vi "setSweepTable.vi"(8 "error in (no error)":errorcluster, 9 "Table(s)":variant, 10 "Channel(s)":variant, 11 "Instrument.LockinAPI in":refnum<class "Instrument.LockinAPI.lvclass">) -> (0 "error out":errorcluster, 3 "Instrument.LockinAPI out":refnum<class "Instrument.LockinAPI.lvclass">)   [LabVIEW 2019, in "Instrument.LockinAPI.lvclass"]
doc: "API to set Sweep Waveform"
uses:
  Instrument.LockinAPI.lvclass
  C:/Users/patrick/Documents/GitHub/Instrument-Framework/lvsrc/Framework/Instrument/Instrument.lvclass
  Typedefs/LockinAPI.Commands--Enum.ctl
  <vilib>/Utility/Data Type/NI_Data Type.lvlib
  Instrument/Instrument.lvclass
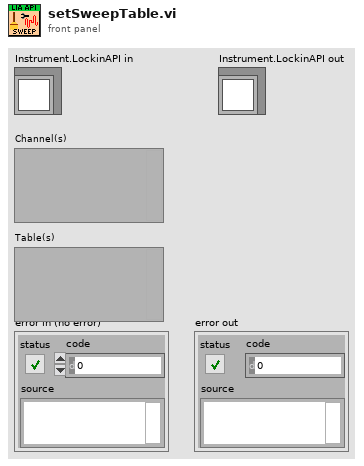
[diagram p1: front panel]
types:
  T1 = cluster{"Sweep Time (s)":dbl, "Initial Wait (s)":dbl, "Return to Start":bool, "Channels":cluster{"Enable?":bool, "Channel":u16, "Start":dbl, "End":dbl, "Pattern":enum16{"Ramp /", "Ramp /\\", "Smooth Ramp _/", "Smooth Ramp _/\\_", "Table"}, "Table":dbl[]}[]}
  T2 = typedef "Instrument.LockinAPI.lvclass/LockinAPI.Commands--Enum.ctl" = enum16{"setAI", "setAO", "setAO_Amplitude", "setAO_DC", "setAO_Frequency", "setAO_Phase", "setAO_Function", "setAO_I+", "setREF", "setREF_Frequency", "setREF_Phase", "setREF_TC", "setREF_Roll-Off", "setDAQ", "setSampling", "setOffset", "setState", "getState", "getAO", "getAI", "getResults", "getSampling", "getAOconfig", "getREFconfig", "setInputGain", "setOutputGain", "getInputGain", "getOutputGain", "setSamplingMode", "getSamplingMode", "setSweep", "setSweepTime", "setSweepTable", "getStatus", "getSweepResults", "getSweepWaveforms", "startSweep", "stopSweep", "setAUX", "getAUX"}
  T3 = cluster{"Enable?":bool, "Channel":u16, "Start":dbl, "End":dbl, "Pattern":enum16{"Ramp /", "Ramp /\\", "Smooth Ramp _/", "Smooth Ramp _/\\_", "Table"}, "Table":dbl[]}[]
  T4 = typedef "NI_Data Type.lvlib/Data Type.ctl" = enum8{"Invalid Type", "Void", "I8", "I16", "I32", "I64", "U8", "U16", "U32", "U64", "Single Float", "Double Float", "Extended Float", "Single Complex", "Double Complex", "Extended Complex", "Enum U8", "Enum U16", "Enum U32", "Enum U64", "Single Float With Unit", "Double Float With Unit", "Extended Float With Unit", "Single Complex with Unit", "Double Complex with Unit", "Extended Complex with Unit", "Boolean", "String", "Path", "Picture", "Tag", "Array", "Cluster", "Variant", "LV Variant", "Waveform", "Timestamp", "Digital Waveform", "Digital Data", "ExpressData", "Refnum", "External Data", "VI", "Poly VI", "LabVIEW Class Instance", "Fixed Point", "Set Collection", "Map Collection"}
  T5 = cluster{"Enable?":bool, "Channel":u16, "Start":dbl, "End":dbl, "Pattern":enum16{"Ramp /", "Ramp /\\", "Smooth Ramp _/", "Smooth Ramp _/\\_", "Table"}, "Table":dbl[]}
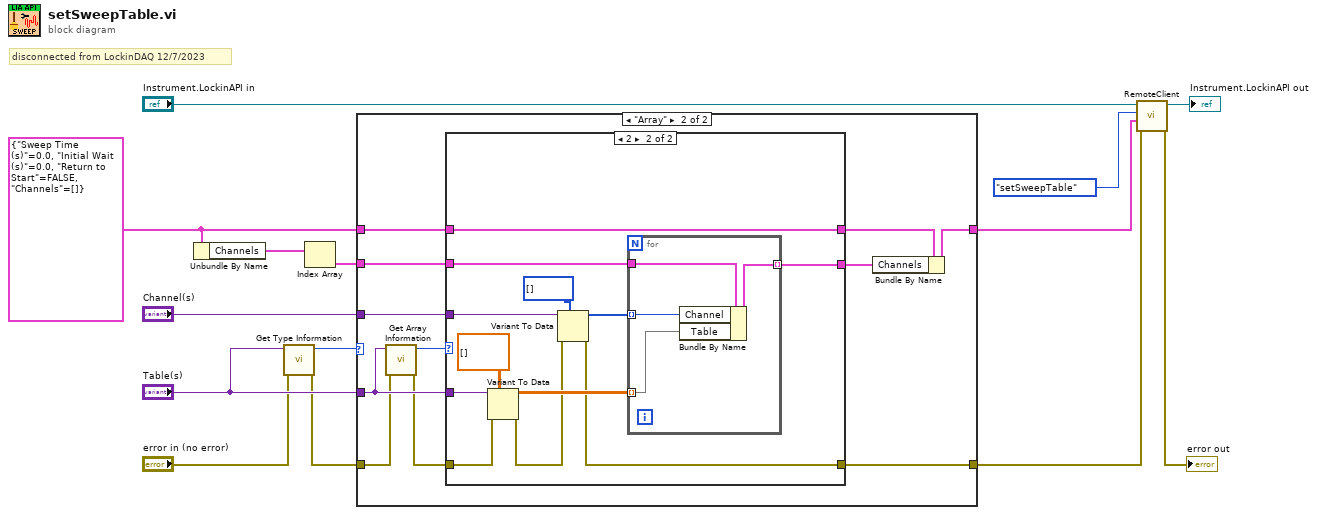
[diagram p0: block diagram]
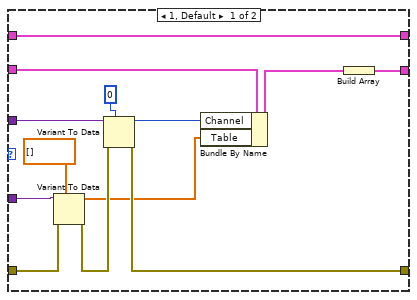
[diagram p3: hidden frame]
diagram:
  w9 = T1 {"Sweep Time (s)"=0.0, "Initial Wait (s)"=0.0, "Return to Start"=FALSE, "Channels"=[]} ("Configure Sweep")
  # "disconnected from LockinDAQ 12/7/2023"
  n1 = Unbundle By Name(w9) -> ("Channels"=w8:T3)
  n2 = call <vilib>:"Get Type Information.vi"("error in (no error)"="error in (no error)", "variant"="Table(s)") -> ("error out"=w3:errorcluster, "type"=w5:T4)  [unwired: 5 in, 3 out]
  n3 = Index Array(array=w8) -> (element=w7:T5)  [unwired: 1 in]
  n4 = case shown="\"Array\"" w5 {
    tunnel: "Channel(s)" -> [_ w27]
    tunnel: w9 -> [w16 w26]
    tunnel: w7 -> [_ w25]
    tunnel: [w16 w19] -> w1
    tunnel: "Table(s)" -> [_ w24]
    tunnel: w3 -> [w15 w22]
    tunnel: [w15 w17] -> w2
    frame "Invalid Type", Default {
    }
    frame "Array" {
      n5 = call <vilib>:"Get Array Information.vi"("error in (no error)"=w22, "variant"=w24) -> ("error out"=w18:errorcluster, "number of dimensions"=w23:i32)  [unwired: 6 in, 2 out]
      n6 = case shown="2" w23 {
        tunnel: w27 -> [w32 w45]
        tunnel: w26 -> [w39 w51]
        tunnel: w25 -> [w40 w52]
        tunnel: [w39 w51] -> w21
        tunnel: [w38 w50] -> w20
        tunnel: w24 -> [w36 w47]
        tunnel: w18 -> [w35 w46]
        tunnel: [w29 w41] -> w17
        frame 1, Default {
          n7 = Variant To Data(error in=w35, type=dbl[] [] ("Pattern"), Variant=w36) -> (data=w28:dbl[], error out=w30:errorcluster)
          n8 = Variant To Data(error in=w30, type=0 ("Channel"), Variant=w32) -> (data=w31:i32, error out=w29:errorcluster)
          n9 = Bundle By Name(cluster=w40, "Channel"=w31, "Table"=w28) -> (w34:T5)
          n10 = Build Array(w34) -> (w38:T3)
        }
        frame 2 {
          n11 = Variant To Data(error in=w46, type=dbl[][] [] ("Pattern"), Variant=w47) -> (data=w48:dbl[][], error out=w42:errorcluster)
          n12 = Variant To Data(error in=w42, type=i32[] [] ("Channel"), Variant=w45) -> (data=w43:i32[], error out=w41:errorcluster)
          n13 = for {
            tunnel: [w53] -> w50 mode=indexing
            tunnel: w48 -> [w56] mode=indexing
            tunnel: w43 -> [w55] mode=indexing
            tunnel: w52 -> [w54]
            n14 = Bundle By Name(cluster=w54, "Channel"=w55, "Table"=w56) -> (w53:T5)
          }
        }
      }
      n15 = Bundle By Name(cluster=w21, "Channels"=w20) -> (w19:T1)
    }
  }
  n16 = call "RemoteClient.vi"("error in (no error)"=w2, "Data in"=w1, "Command in"=LockinAPI.Commands--Enum."setSweepTable" ("Command"), "Instrument in"="Instrument.LockinAPI in") -> ("error out"=→"error out":errorcluster, "Instrument out"=→"Instrument.LockinAPI out":refnum<class "Instrument.LockinAPI.lvclass">)  [unwired: 4 in, 2 out]
